vi "PID_Control_Dashboard.vi"() -> ()   [LabVIEW 2022 SP3]
uses:
  <vilib>/Instr/_visa.llb/VISA Configure Serial Port (Instr).vi
panel:
  out "ball position":dbl(graph)
  in  "stop":bool
  in  "baud rate (9600)":u32=9600
  in  "VISA resource name":refnum<visa-resource-name>
  out "Ball position":dbl(slide) scale=0.0..40.0
  in  "Setpoint":bool
  in  "Manual setpoint":dbl(slide) scale=0.0..40.0
  out "Hand position":dbl(slide) scale=0.0..40.0
  out "Waveform Chart":dbl(graph)
  out "HAND":dbl
  out "BALL":dbl
  out "Error":dbl
  out "SetPoint":dbl
  out "PWM":dbl
  out "PWM 2":dbl
  # "By Hand"
  # "manual"
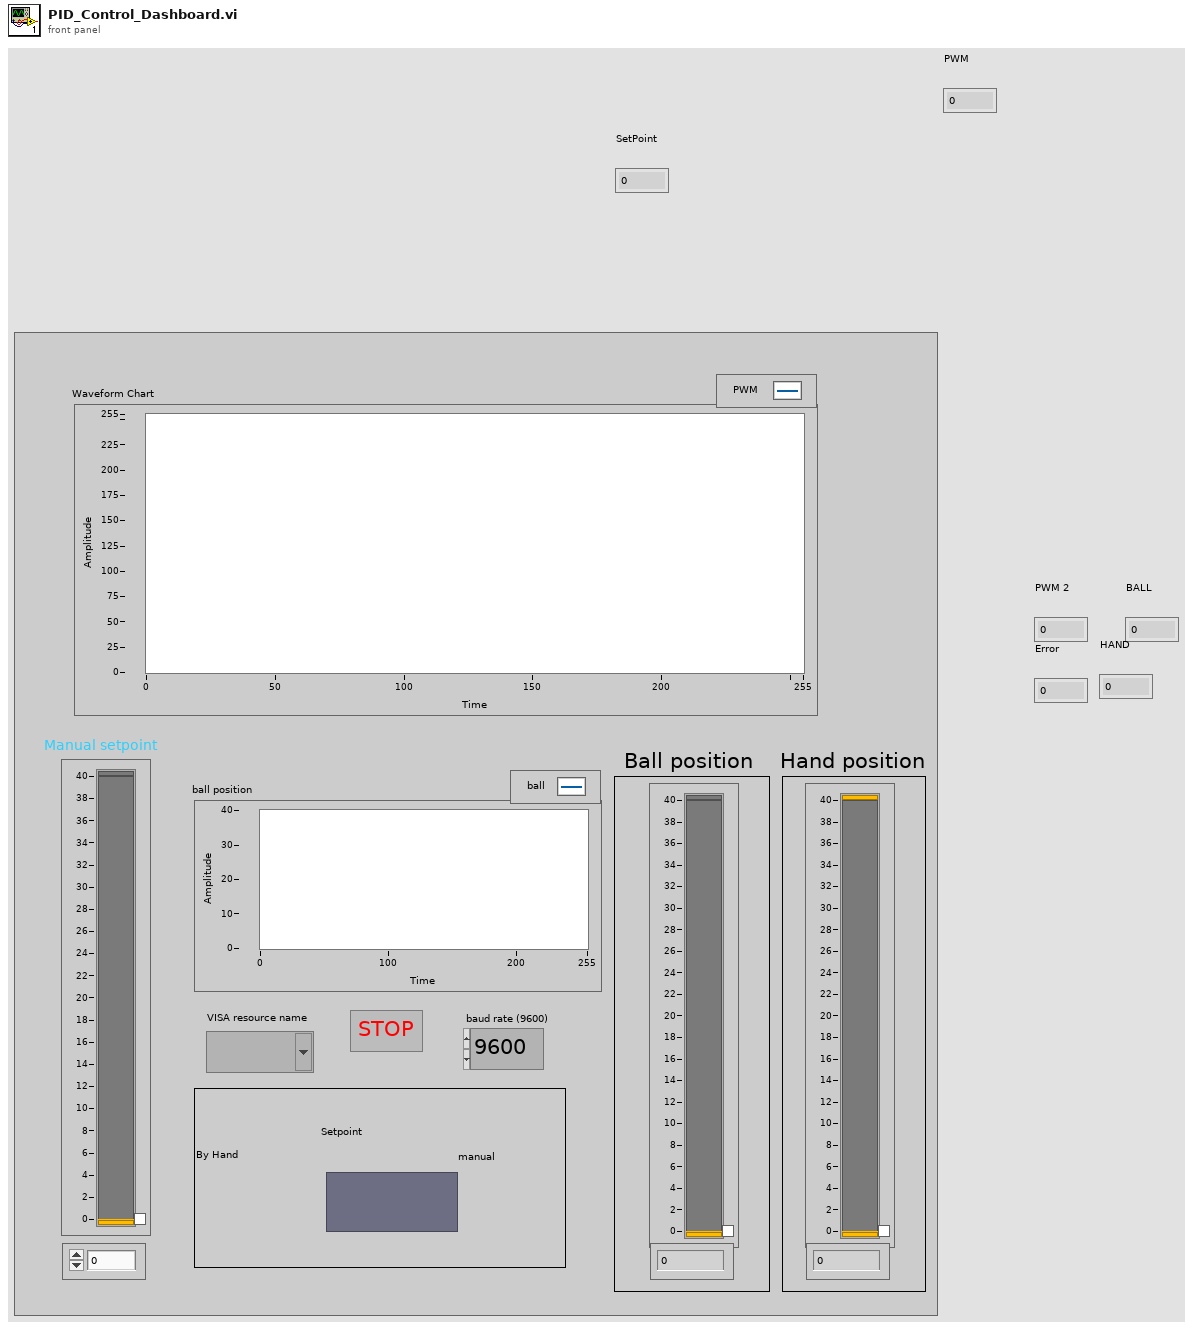
[diagram p1: front panel]
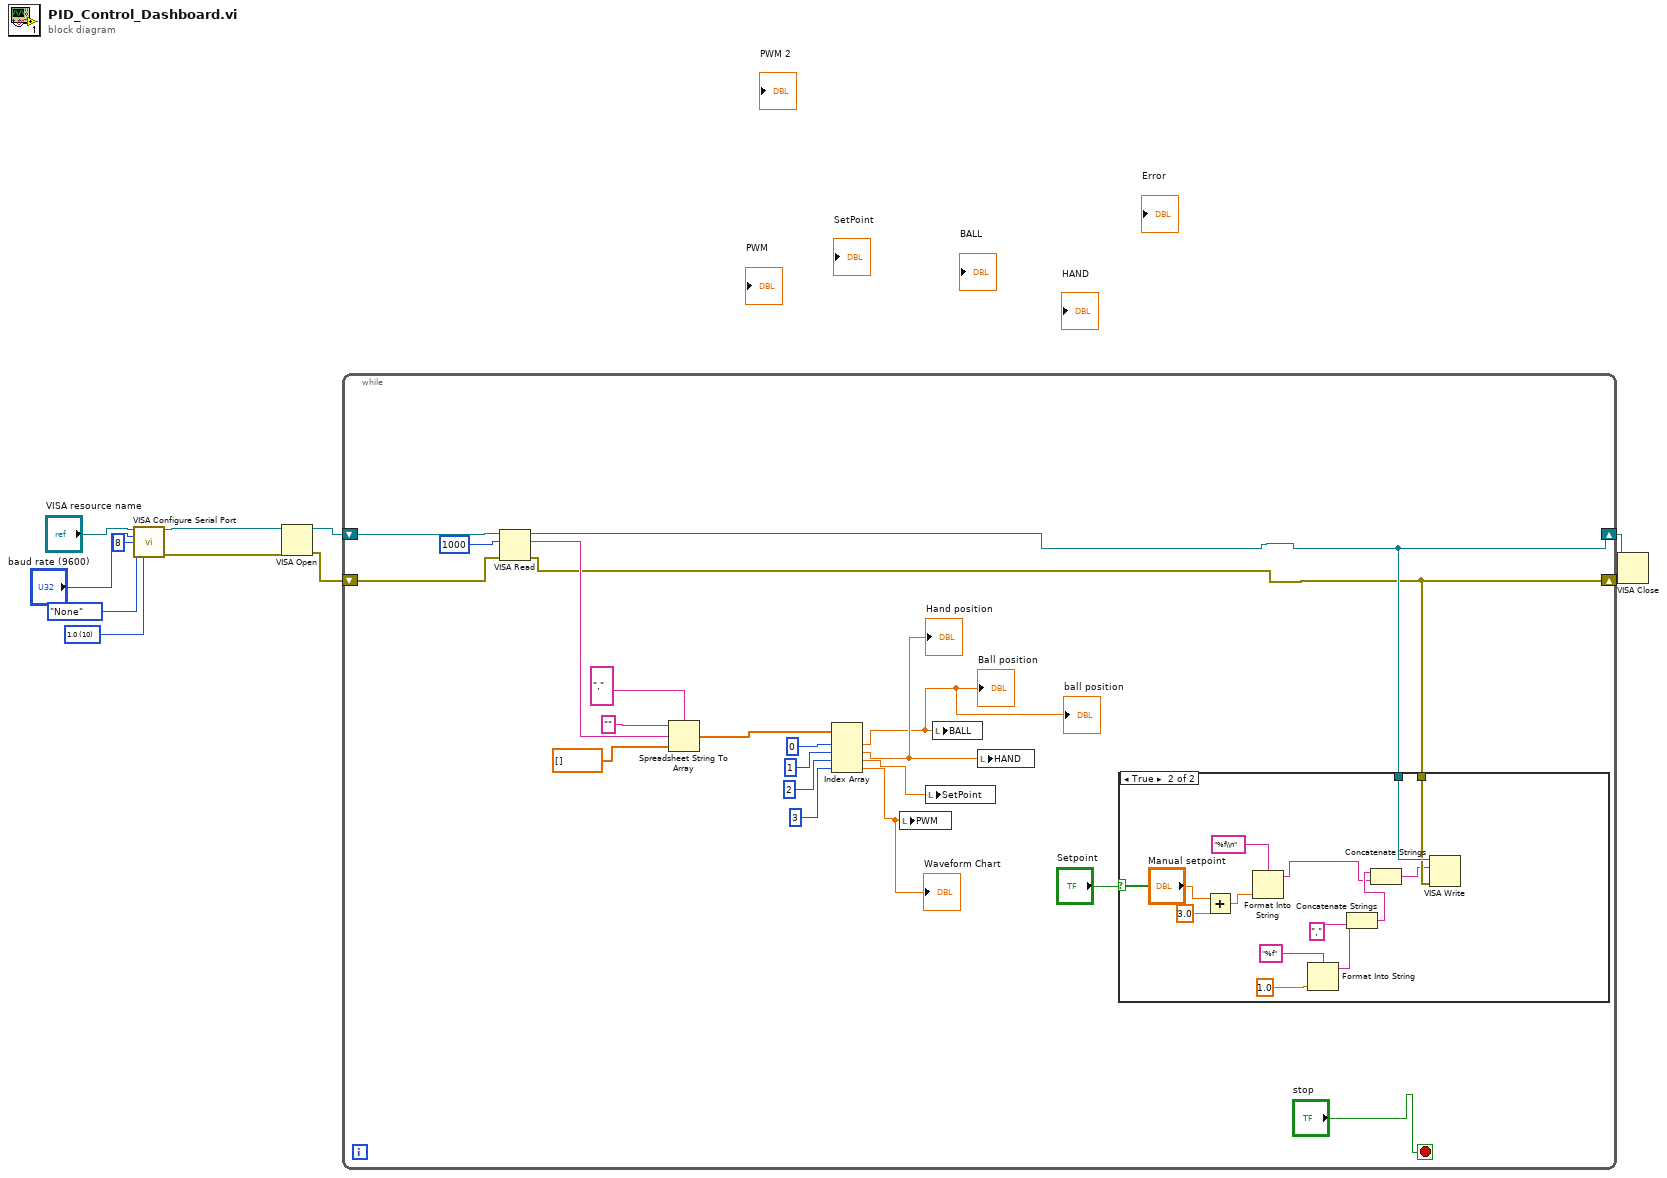
[diagram p0: block diagram]
diagram:
  w9 = u16 10 items=["1.0"=10, "1.5"=15, "2.0"=20] ("stop bits (10: 1 bit)")
  n1 = call-poly "VISA Configure Serial Port"("VISA resource name"="VISA resource name", "baud rate (9600)"="baud rate (9600)", "data bits (8)"=u16 8, "parity (0:none)"=enum16{"None", "Odd", "Even", "Mark", "Space"}."None", "stop bits (10: 1 bit)"=w9) -> ("VISA resource name out"=w8:refnum<visa-resource-name>, "error out"=w7:errorcluster)  [unwired: 9 in]
  n2 = VISA Open(error in (no error)=w7, VISA resource name=w8) -> (VISA resource name=w6:refnum<visa-resource-name>, error out=w5:errorcluster)  [unwired: 3 in]
  n3 = while {
    shift-right: [w13] -> w4
    shift-left: w6 -> [w18]
    shift-right: [w12] -> w3
    shift-left: w5 -> [w17]
    stop <- "stop" stop-if-true
    n4 = VISA Read(VISA resource name=w18, byte count=u32 1000, error in (no error)=w17) -> (VISA resource name out=w13:refnum<visa-resource-name>, read buffer=w30:string, error out=w12:errorcluster)  [unwired: 1 out]
    n5 = Spreadsheet String To Array(delimiter (Tab)=",", format string="", spreadsheet string=w30, array type (2D Dbl)=dbl[] []) -> (array=w28:dbl[])
    n6 = Index Array(array=w28, index #1=0 ("index"), index #2=1 ("index"), index #3=2 ("index"), index #4=3 ("index")) -> (element #1=w14:dbl, element #2=w16:dbl, element #3=w23:dbl, element #4=w20:dbl)
    "Waveform Chart" <- w20
    "Hand position" <- w16
    "Ball position" <- w14
    "ball position" <- w14
    n7 = local write "PWM"(w20) -> ()
    n8 = local write "SetPoint"(w23) -> ()
    n9 = local write "BALL"(w14) -> ()
    n10 = local write "HAND"(w16) -> ()
    n11 = case shown="True" "Setpoint" {
      tunnel: w13 -> [_ w43]
      tunnel: w12 -> [_ w42]
      frame False {
      }
      frame True {
        n12 = Add(x="Manual setpoint", y=3.0) -> (x+y=w33:dbl)
        n13 = Format Into String(format string="%f\\n", w33) -> (resulting string=w36:string)  [unwired: 2 in, 1 out]
        n14 = Format Into String(format string="%f", 1.0 ("input 1")) -> (resulting string=w39:string)  [unwired: 2 in, 1 out]
        n15 = Concatenate Strings(w39, "," ("string")) -> (w37:string)
        n16 = Concatenate Strings(w37, w36) -> (w35:string)
        n17 = VISA Write(VISA resource name=w43, write buffer=w35, error in (no error)=w42) -> ()  [unwired: 3 out]
      }
    }
  }
  n18 = VISA Close(VISA resource name=w4, error in (no error)=w3) -> ()  [unwired: 1 out]
